vi "Laboratory_practice13.vi"() -> ()   [LabVIEW 2021]
panel:
  in  "rate":dbl=5000.0
  in  "number of samples":i32=100
  out "data":dynamicdata(graph)
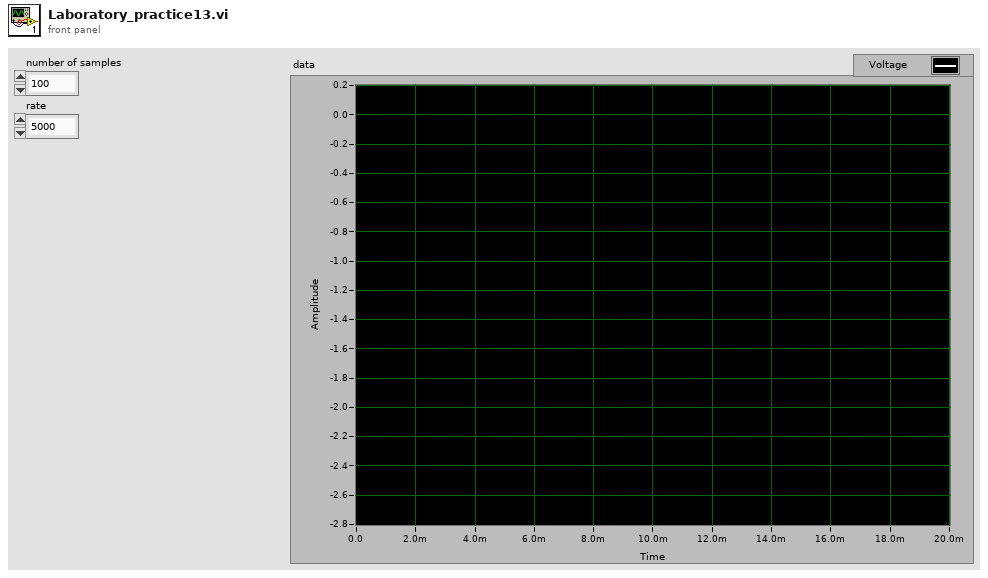
[diagram p1: front panel]
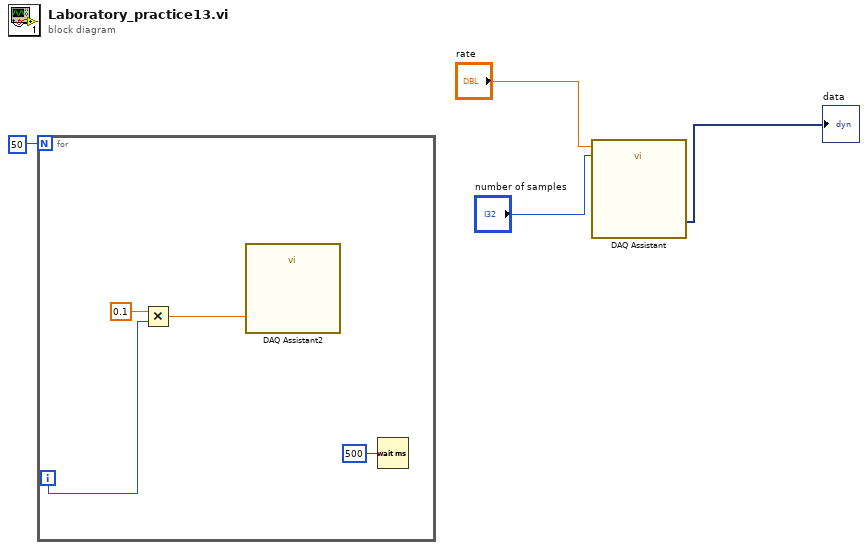
[diagram p0: block diagram]
diagram:
  n1 = for {
    N: 50 -> [_]
    i -> [w6]
    n2 = Multiply(x=0.1, y=w6) -> (x*y=w5:dbl)
    n3 = call "DAQ Assistant2"("data"=w5) -> ()  [unwired: 17 in, 2 out]
    n4 = Wait (ms)(milliseconds to wait=u32 500) -> ()  [unwired: 1 out]
  }
  n5 = call "DAQ Assistant"("rate"="rate", "number of samples"="number of samples") -> ("data"=→"data":dynamicdata)  [unwired: 15 in, 2 out]
